vi "Create.vi"(8 "error in (no error)":errorcluster, 10 "configuration file path":path) -> (0 "error out":errorcluster, 3 "Configuration Manager out":refnum<class "Configuration Manager.lvclass">)   [LabVIEW 2020, in "Configuration Manager.lvclass"]
uses:
  Configuration Manager.lvclass
  Configuration Manager.lvclass/Configuration Manager.ctl
  <vilib>/Utility/config.llb/NI_LVConfig.lvlib
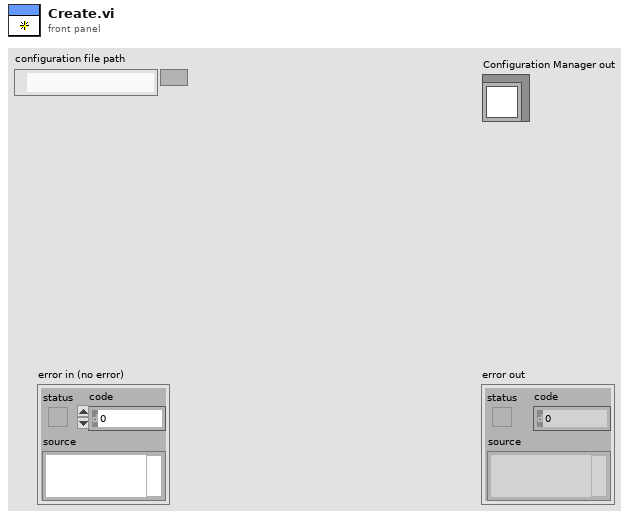
[diagram p1: front panel]
types:
  T1 = typedef "NI_LVConfig.lvlib/Config Data RefNum.ctl" = refnum<k1>
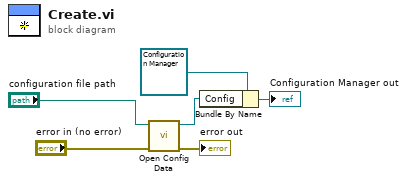
[diagram p0: block diagram]
diagram:
  n1 = call <vilib>:"Open Config Data.vi"("error in (no error)"="error in (no error)", "configuration file path"="configuration file path") -> ("error out"=→"error out":errorcluster, "refnum"=w1:T1)  [unwired: 7 in, 1 out]
  n2 = Bundle By Name(cluster=refnum<class "Configuration Manager.lvclass"> refnum ("Configuration Manager in"), "Config"=w1) -> (→"Configuration Manager out":refnum<class "Configuration Manager.lvclass">)
